vi "Drive Test 2016.vi"(10 "Pilot-CoPilot Controls":T1) -> ()   [LabVIEW 2015]
uses:
  Robot Control Outputs 2016.ctl
  <vilib>/Rock Robotics/WPI/Solenoid/WPI_SolenoidValue.ctl
  Global Variables/refnum names.vi
  <vilib>/Rock Robotics/WPI/Solenoid/WPI_SolenoidSetEnum.vi
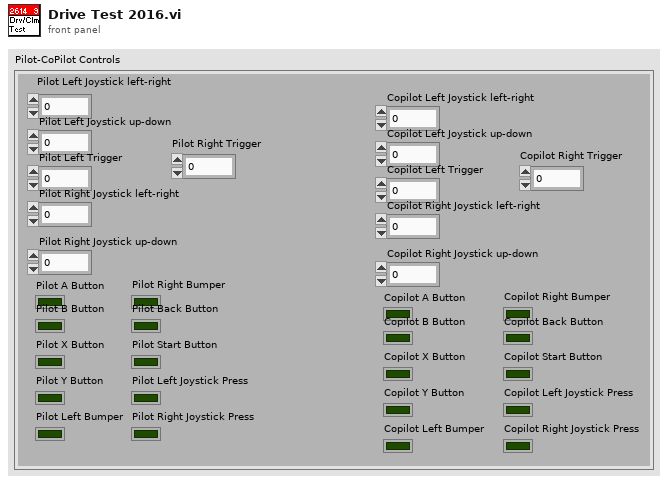
[diagram p1: front panel]
types:
  T1 = typedef "Robot Control Outputs 2016.ctl" = cluster{"Pilot Left Joystick left-right":dbl, "Pilot Left Joystick up-down":dbl, "Pilot A Button":bool, "Pilot B Button":bool, "Pilot X Button":bool, "Pilot Y Button":bool, "Pilot Left Bumper":bool, "Pilot Right Bumper":bool, "Pilot Back Button":bool, "Pilot Start Button":bool, "Pilot Left Joystick Press":bool, "Pilot Right Joystick Press":bool, "Pilot Left Trigger":dbl, "Pilot Right Joystick left-right":dbl, "Pilot Right Joystick up-down":dbl, "Pilot Right Trigger":dbl, "Copilot Left Joystick left-right":dbl, "Copilot Left Joystick up-down":dbl, "Copilot A Button":bool, "Copilot B Button":bool, "Copilot X Button":bool, "Copilot Y Button":bool, "Copilot Left Bumper":bool, "Copilot Right Bumper":bool, "Copilot Back Button":bool, "Copilot Start Button":bool, "Copilot Left Joystick Press":bool, "Copilot Right Joystick Press":bool, "Copilot Left Trigger":dbl, "Copilot Right Joystick left-right":dbl, "Copilot Right Joystick up-down":dbl, "Copilot Right Trigger":dbl}
  T2 = typedef "WPI_SolenoidValue.ctl" = enum16{"Off", "On", "Forward", "Reverse"}
  T3 = typedef "WPI_MotorControlDeviceRef.ctl" = cluster{"DeviceStatus":errorcluster, "Type":T4, "PWM":cluster{"PWM Channel":T5, "DeadBand":T6}, "CAN":cluster{"Device Number":u8, "Control Mode":T7, "Semaphore":T8, "Max Vout":dbl, "TalonSRX Control Mode":T9}, "Invert":bool}
  T4 = typedef "WPI_MotorControlType.ctl" = enum16{"PWM", "CAN", "CANTalonSRX"}
  T5 = typedef "FPGA_DIOPWMChannel.ctl" = enum8{"PWM 0", "PWM 1", "PWM 2", "PWM 3", "PWM 4", "PWM 5", "PWM 6", "PWM 7", "PWM 8", "PWM 9", "PWM MXP 0", "PWM MXP 1", "PWM MXP 2", "PWM MXP 3", "PWM MXP 4", "PWM MXP 5", "PWM MXP 6", "PWM MXP 7", "PWM MXP 8", "PWM MXP 9", "Invalid"}
  T6 = typedef "WPI_PWMDeadband.ctl" = cluster{"Name":string, "maxPositivePwm":i32, "minPositivePwm":i32, "centerPwm":i32, "maxNegativePwm":i32, "minNegativePwm":i32, "angularRange":u16}
  T7 = typedef "WPI_CANJaguar_ControlMode.ctl" = enum8{"Percent VBus", "Current", "Speed", "Position", "Voltage"}
  T8 = typedef "Semaphore RefNum" = refnum<k1>
  T9 = typedef "WPI_CANTalonSRX_APIControlMode.ctl" = enum8{"Percent VBus", "Speed", "Position", "Slave", "Unchanged / Invalid", "Voltage Compensation", "Current", "Motion Profile"}
  T10 = typedef "WPI_CANTalonSRX_GlobalStatus.ctl" = cluster{"Applied Throttle":dbl, "Module Enabled":bool, "CAN Error":errorcluster, "Closed Loop Error":dbl, "Forward Limit Switch Closed":bool, "Reverse Limit Switch Closed":bool, "Sensor Position":dbl, "Sensor Velocity":dbl, "Current":dbl, "Sticky Fault - Over Temp":bool, "Sticky Fault - Under Voltage":bool, "Sticky Fault - Forward Limit":bool, "Sticky Fault - Reverse Limit":bool, "Sticky Fault - Forward Soft Limit":bool, "Sticky Fault - Reverse Soft Limit":bool, "Brake is Enabled":bool, "Encoder Position":dbl, "Encoder Velocity":dbl, "Encoder Index Count":dbl, "Encoder A Pin State":bool, "Encoder B Pin State":bool, "Encoder Index Pin State":bool, "Analog In":dbl, "Analog In Velocity":dbl, "Temperature (C)":dbl, "Battery Voltage":dbl, "Control 5 Is Supported":bool, "Current Profile Slot Select":dbl, "Pos Div 8":bool, "Vel Div 4":bool, "Pulse Width Position":i32, "Pulse Width Velocity":i32, "Pulse Width Rise To Rise (us)":i32, "Pulse Width Rise To Fall (us)":i32, "Mot Prof Active Is Under Run":bool, "Mot Prof Active Has Under Run":bool, "Mot Prof Active Is Last":bool, "Mot Prof Active Velocity Only":bool, "Mot Prof Active Is Valid":bool, "Mot Prof Buffer Is Full":bool, "Mot Prof Active Profile Slot Select":i32, "Mot Prof NextID":i32, "Mot Prof Count":i32, "Mot Prof Active Velocity":dbl, "Mot Prof Active Position":dbl, "Mot Prof Output Enable":i32}
  T11 = typedef "WPI_SolenoidDevRef.ctl" = cluster{"DevStatus":errorcluster, "Pneumatics Control Module":u8, "Forward Solenoid Channel":T12, "Reverse Solenoid Channel":T12}
  T12 = typedef "WPI_SolenoidChannel.ctl" = enum8{"Solenoid 0", "Solenoid 1", "Solenoid 2", "Solenoid 3", "Solenoid 4", "Solenoid 5", "Solenoid 6", "Solenoid 7", "Invalid"}
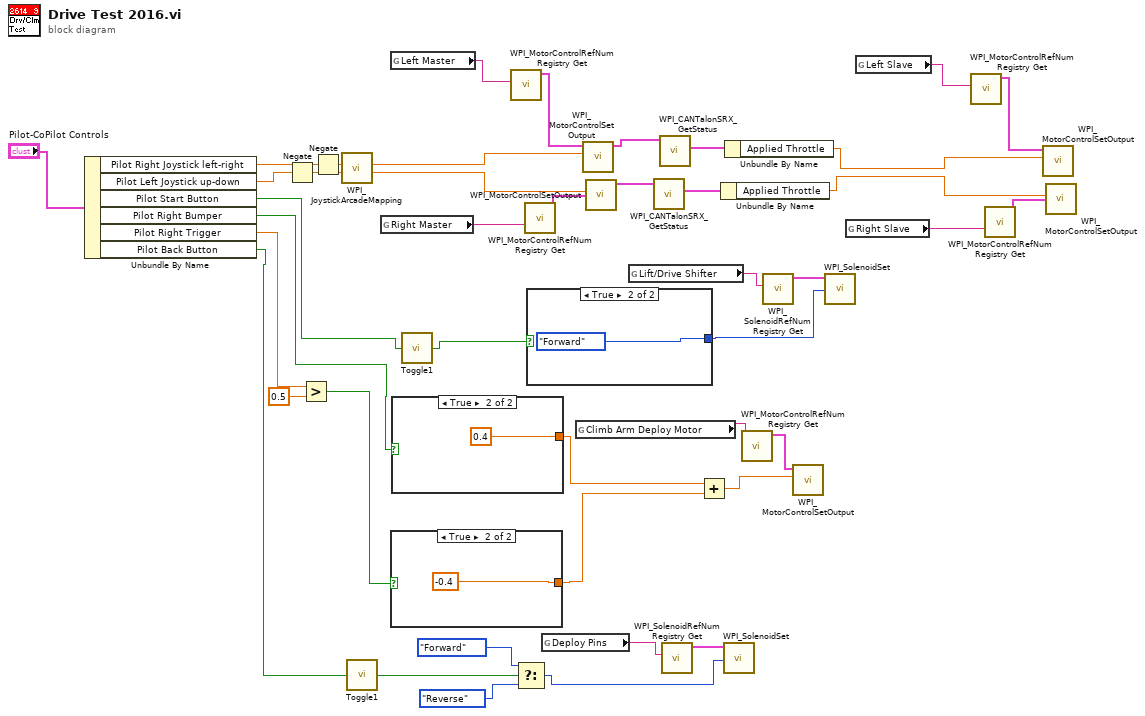
[diagram p0: block diagram]
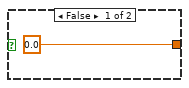
[diagram p2: hidden frame]
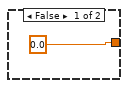
[diagram p3: hidden frame]
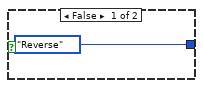
[diagram p4: hidden frame]
diagram:
  n1 = Unbundle By Name("Pilot-CoPilot Controls") -> ("Pilot Right Joystick left-right"=w41:dbl, "Pilot Left Joystick up-down"=w40:dbl, "Pilot Start Button"=w33:bool, "Pilot Right Bumper"=w23:bool, "Pilot Right Trigger"=w28:dbl, "Pilot Back Button"=w17:bool)
  n2 = Negate(x=w40) -> (-x=w19:dbl)
  n3 = Greater?(x=w28, y=0.5) -> (0:w24:bool)
  n4 = Negate(x=w41) -> (-x=w18:dbl)
  n5 = call <vilib>:"WPI_JoystickArcadeMapping.vi"("Y axis value"=w19, "X axis value"=w18) -> ("Right Motor Value"=w38:dbl, "Left Motor Value"=w39:dbl)  [unwired: 8 in]
  n6 = call "Toggle1.vi"("Boolean"=w17) -> ("Driver Switch 2"=w14:bool)
  n7 = global read "refnum names.vi" "Right Master"() -> (w37:string)
  n8 = global read "refnum names.vi" "Left Master"() -> (w34:string)
  n9 = case shown="True" w24 {
    tunnel: [0.0 -0.4] -> w21
    frame False {
    }
    frame True {
    }
  }
  n10 = case shown="True" w23 {
    tunnel: [0.0 0.4] -> w22
    frame False {
    }
    frame True {
    }
  }
  n11 = call "Toggle1.vi"("Boolean"=w33) -> ("Driver Switch 2"=w32:bool)
  n12 = call <vilib>:"WPI_MotorControlRefNum Registry Get.vi"("refnum name"=w34) -> ("MotorControlDevRef"=w35:T3)  [unwired: 9 in, 1 out]
  n13 = Select(t=WPI_SolenoidValue."Forward" ("Value"), s=w14, f=WPI_SolenoidValue."Reverse" ("Value")) -> (s? t:f=w11:T2)
  n14 = call <vilib>:"WPI_MotorControlRefNum Registry Get.vi"("refnum name"=w37) -> ("MotorControlDevRef"=w36:T3)  [unwired: 9 in, 1 out]
  n15 = case shown="True" w32 {
    tunnel: [WPI_SolenoidValue."Reverse" ("Value") WPI_SolenoidValue."Forward" ("Value")] -> w29
    frame False {
    }
    frame True {
    }
  }
  n16 = global read "refnum names.vi" "Deploy Pins"() -> (w12:string)
  n17 = global read "refnum names.vi" "Climb Arm Deploy Motor"() -> (w26:string)
  n18 = call <vilib>:"WPI_MotorControlSetOutput.vi"("Output"=w39, "MotorControlDevRef"=w35) -> ("MotorControlDevRef"=w10:T3)  [unwired: 7 in, 2 out]
  n19 = call <vilib>:"WPI_MotorControlSetOutput.vi"("Output"=w38, "MotorControlDevRef"=w36) -> ("MotorControlDevRef"=w9:T3)  [unwired: 7 in, 2 out]
  n20 = global read "refnum names.vi" "Lift/Drive Shifter"() -> (w31:string)
  n21 = call <vilib>:"WPI_CANTalonSRX_GetStatus.vi"("CAN Talon SRX Ref"=w9) -> ("Talon SRX Status"=w7:T10)  [unwired: 8 in, 2 out]
  n22 = call <vilib>:"WPI_CANTalonSRX_GetStatus.vi"("CAN Talon SRX Ref"=w10) -> ("Talon SRX Status"=w8:T10)  [unwired: 8 in, 2 out]
  n23 = call <vilib>:"WPI_SolenoidRefNum Registry Get.vi"("refnum name"=w12) -> ("SolenoidDevRef"=w13:T11)  [unwired: 9 in, 1 out]
  n24 = Add(x=w22, y=w21) -> (x+y=w20:dbl)
  n25 = Unbundle By Name(w7) -> ("Applied Throttle"=w1:dbl)
  n26 = call-poly <vilib>:"WPI_SolenoidSet.vi"("Value"=w11, "SolenoidDevRef"=w13) -> ()  [unwired: 8 in, 2 out]
  n27 = Unbundle By Name(w8) -> ("Applied Throttle"=w2:dbl)
  n28 = call <vilib>:"WPI_MotorControlRefNum Registry Get.vi"("refnum name"=w26) -> ("MotorControlDevRef"=w25:T3)  [unwired: 9 in, 1 out]
  n29 = call <vilib>:"WPI_SolenoidRefNum Registry Get.vi"("refnum name"=w31) -> ("SolenoidDevRef"=w30:T11)  [unwired: 9 in, 1 out]
  n30 = call <vilib>:"WPI_MotorControlSetOutput.vi"("Output"=w20, "MotorControlDevRef"=w25) -> ()  [unwired: 7 in, 3 out]
  n31 = call-poly <vilib>:"WPI_SolenoidSet.vi"("Value"=w29, "SolenoidDevRef"=w30) -> ()  [unwired: 8 in, 2 out]
  n32 = global read "refnum names.vi" "Right Slave"() -> (w3:string)
  n33 = global read "refnum names.vi" "Left Slave"() -> (w6:string)
  n34 = call <vilib>:"WPI_MotorControlRefNum Registry Get.vi"("refnum name"=w6) -> ("MotorControlDevRef"=w5:T3)  [unwired: 9 in, 1 out]
  n35 = call <vilib>:"WPI_MotorControlRefNum Registry Get.vi"("refnum name"=w3) -> ("MotorControlDevRef"=w4:T3)  [unwired: 9 in, 1 out]
  n36 = call <vilib>:"WPI_MotorControlSetOutput.vi"("Output"=w2, "MotorControlDevRef"=w5) -> ()  [unwired: 7 in, 3 out]
  n37 = call <vilib>:"WPI_MotorControlSetOutput.vi"("Output"=w1, "MotorControlDevRef"=w4) -> ()  [unwired: 7 in, 3 out]
